vi "Write Data.vi"(8 "error in":errorcluster, 10 "Data":refnum<class "Data.lvclass">, 11 "Send Data Msg in":refnum<class "Send Data Msg.lvclass">) -> (0 "error out":errorcluster, 3 "Send Data Msg out":refnum<class "Send Data Msg.lvclass">)   [LabVIEW 2014, in "Send Data Msg.lvclass"]
uses:
  Send Data Msg.lvclass
  Data/Data.lvlibp/Data.lvclass
  Send Data Msg.lvclass/Send Data Msg.ctl
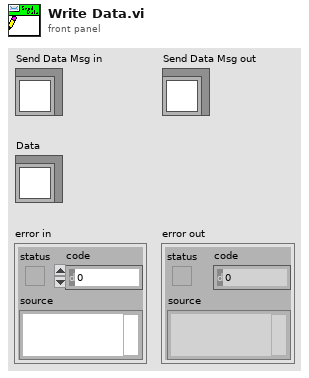
[diagram p1: front panel]
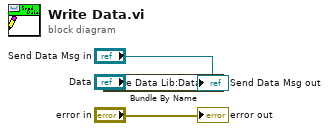
[diagram p0: block diagram]
diagram:
  n1 = Bundle By Name(cluster="Send Data Msg in", "Base Data Lib:Data"="Data") -> (→"Send Data Msg out":refnum<class "Send Data Msg.lvclass">)
  "error out" <- "error in"
